vi "Tree_Sync Drag and Drop.vi"(9 "Value on Drag":string[](array[string]), 10 "TreeControl in":refnum<vi>, 11 "Tree Ref Array":refnum<vi>[](array[refnum])) -> ()   [LabVIEW 2023]
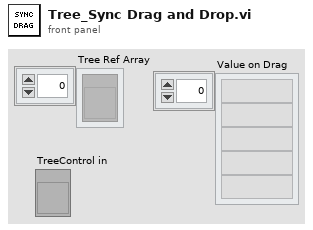
[diagram p1: front panel]
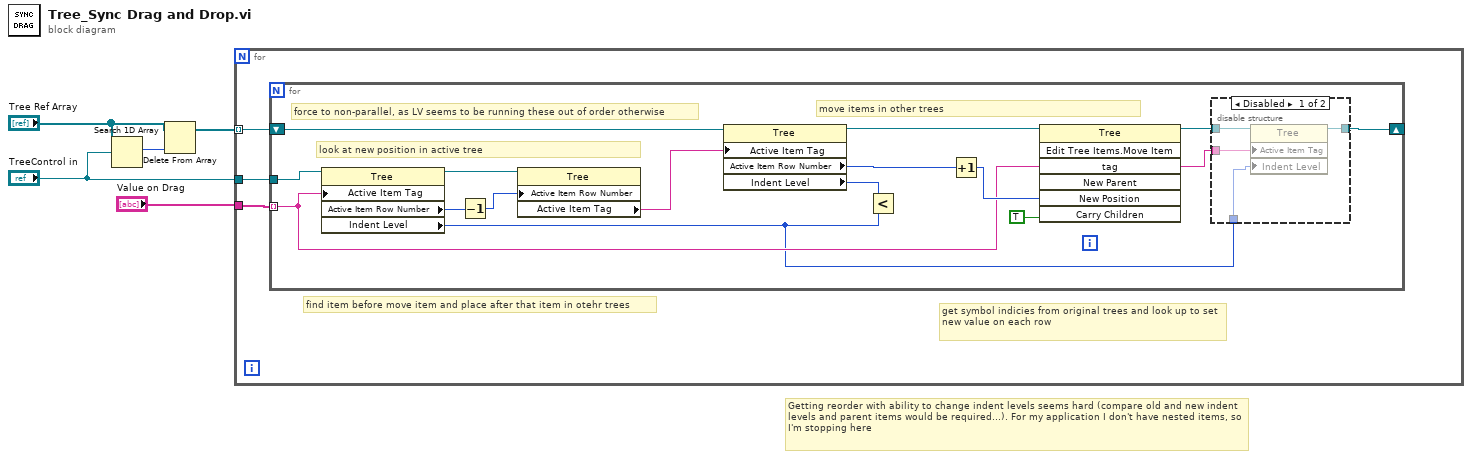
[diagram p0: block diagram]
diagram:
  # "Getting reorder with ability to change indent levels seems hard (compare old and new indent levels and parent items would be required...). For my application I don't have nested items, so I'm stopping here"
  n1 = Search 1D Array(1D array="Tree Ref Array", element="TreeControl in") -> (index of element=w4:i32)  [unwired: 1 in]
  n2 = Delete From Array(array="Tree Ref Array", index=w4) -> (array with subset deleted=w5:refnum<vi>[])  [unwired: 1 in, 1 out]
  n3 = for {
    tunnel: w5 -> [w8] mode=indexing
    tunnel: "Value on Drag" -> [w7]
    tunnel: "TreeControl in" -> [w6]
    # "find item before move item and place after that item in otehr trees"
    # "get symbol indicies from original trees and look up to set new value on each row"
    n4 = for {
      tunnel: w7 -> [w11] mode=indexing
      tunnel: w6 -> [w16]
      shift-right: [w12] -> _
      shift-left: w8 -> [w20]
      # "move items in other trees"
      # "look at new position in active tree"
      # "force to non-parallel, as LV seems to be running these out of order otherwise"
      n5 = property class="Tree"(reference=w16, "Active Item Tag"=w11) -> (reference out=w23:refnum<vi>, "Active Item Row Number"=w22:i32, "Indent Level"=w9:i32)  [unwired: 1 in, 1 out]
      n6 = Decrement(x=w22) -> (x-1=w21:i32)
      n7 = property class="Tree"(reference=w23, "Active Item Row Number"=w21) -> ("Active Item Tag"=w19:string)  [unwired: 1 in, 2 out]
      n8 = property class="Tree"(reference=w20, "Active Item Tag"=w19) -> (reference out=w17:refnum<vi>, "Active Item Row Number"=w18:i32, "Indent Level"=w10:i32)  [unwired: 1 in, 1 out]
      n9 = Less?(x=w10, y=w9) -> ()  [unwired: 1 out]
      n10 = Increment(x=w18) -> (x+1=w15:i32)
      n11 = invoke class="Tree" method="Edit Tree Items.Move Item"(reference=w17, "tag"=w11, "New Position"=w15, "Carry Children"=TRUE ("Carry Children?")) -> (reference out=w13:refnum<vi>)  [unwired: 3 in, 6 out]
      n12 = disable-structure shown="Disabled" {
        disable-tunnel: w13 -> [w27 w28]
        disable-tunnel: [w26 w28] -> w12
        disable-tunnel: w11 -> [w25 _]
        disable-tunnel: w9 -> [w24 _]
        frame Disabled {
          n13 = property class="Tree"(reference=w27, "Active Item Tag"=w25, "Indent Level"=w24) -> (reference out=w26:refnum<vi>)  [unwired: 1 in, 1 out]
        }
        frame Enabled {
        }
      }
    }
  }
